vi "Prepare.vi"(8 "error in (no error)":errorcluster, 11 "Pizza in":refnum<class "Pizza.lvclass">) -> (0 "error out":errorcluster, 3 "Pizza out":refnum<class "Pizza.lvclass">)   [LabVIEW 2020, in "FactoryMethod.lvlib" / "PizzaFactoryMethod.lvlib" / "Pizza.lvclass"]
uses:
  Pizza.lvclass
  <vilib>/Utility/error.llb/whitespace.ctl
  Pizza.lvclass/Pizza.ctl
  Private/Property/name/Read name.vi
  Private/Property/dough/Read dough.vi
  Private/Property/sauce/Read sauce.vi
  Private/Property/toppings/Read toppings.vi
  Support/Class/ConsoleOutput.lvclass
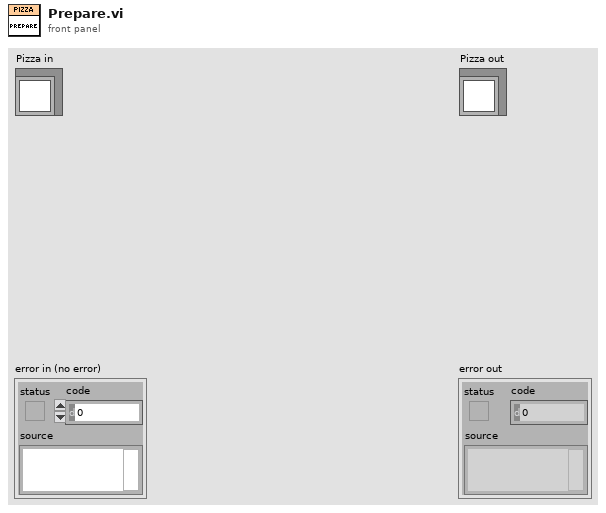
[diagram p1: front panel]
types:
  T1 = typedef "whitespace.ctl" = u16
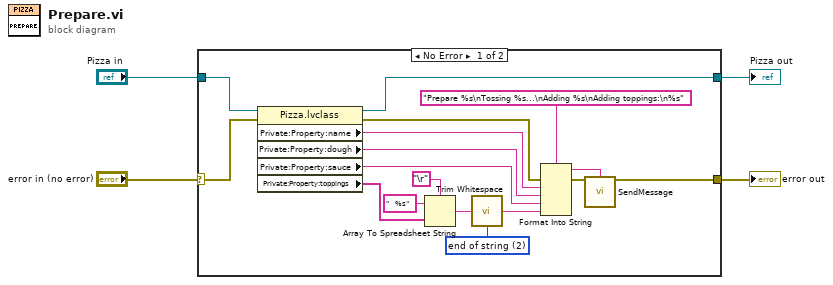
[diagram p0: block diagram]
diagram:
  n1 = case shown="No Error" "error in (no error)" {
    selector: "error in (no error)" -> [w20 w23]
    tunnel: [w11 w23] -> w3
    tunnel: [w13 w22] -> w1
    tunnel: "Pizza in" -> [w21 w22]
    frame No Error {
      w5 = T1 2 items=["both", "start of string", "end of string"] ("location (both)")
      n2 = property class="Pizza.lvclass"(reference=w21, error in=w20) -> (reference out=w13:refnum<class "Pizza.lvclass">, error out=w14:errorcluster, "Private:Property:name"=w17:string, "Private:Property:dough"=w16:string, "Private:Property:sauce"=w15:string, "Private:Property:toppings"=w19:string[])
      n3 = Array To Spreadsheet String(delimiter (Tab)="\r", array=w19, 3:"   %s" ("string")) -> (spreadsheet string=w7:string)
      n4 = call <vilib>:"Trim Whitespace.vi"("string"=w7, "location (both)"=w5) -> ("trimmed string"=w6:string)
      n5 = Format Into String(format string="Prepare %s\nTossing %s...\nAdding %s\nAdding toppings:\n%s" ("string"), error in=w14, w17, w16, w15, w6) -> (resulting string=w10:string, error out=w12:errorcluster)  [unwired: 1 in]
      n6 = call "SendMessage.vi"("Message"=w10, "error in (no error)"=w12) -> ("error out"=w11:errorcluster)  [unwired: 13 in]
    }
    frame Error {
    }
  }
  "error out" <- w3
  "Pizza out" <- w1
